vi "Formatdata.vi"() -> ()   [LabVIEW 2022 SP3, in "Switch_Keysight_34934A.lvlib" / "Switch_Keysight_34934A.lvclass"]
uses:
  Switch_Keysight_34934A.lvclass
  Components/ViPER.lvlibp/ViPER.lvclass
panel:
  in  "Config 2":T1={"VISA"="USB0::0x0957::0x0507::MY56485422::INSTR", "Slot"=1, "SwitchMap"=[{"Name"="Passive_Tests", "Route"=[], "UnRoute"=[], "Description"="Tests component values unpowered", "Group"="", "IsGroup"=TRUE}, {"Name"="Discharge_C108_C109", "Route"=["M1H:1:6:1", "M1H:1:19:1", "M1L:1:6:1", "M1L:1:19:1"], "UnRoute"=["M1H:1:6:0", "M1H:1:19:0", "M1L:1:6:0", "M1L:1:19:0"], "Description"="Discharge the caps for 3 secs", "Group"="Passive_Tests", "IsGroup"=FALSE}, {"Name"="Capacitors", "Route"=[], "UnRoute"=[], "Description"="Tests Capacitor Values", "Group"="Passive_Tests", "IsGroup"=TRUE}, {"Name"="Connect_LCR", "Route"=["M1H:1:23:1", "M1H:2:24:1", "M1L:1:25:1", "M1L:2:26:1"], "UnRoute"=["M1H:1:23:0", "M1H:2:24:0", "M1L:1:25:0", "M1L:2:26:0"], "Description"="Connect the LCR to the Matrix", "Group"="Capacitors", "IsGroup"=FALSE}, {"Name"="C108_C109", "Route"=["M1H:1:6:1", "M1H:2:6:1", "M1L:1:6:1", "M1L:2:6:1"], "UnRoute"=["M1H:1:6:0", "M1H:2:6:0", "M1L:1:6:0", "M1L:2:6:0"], "Description"="C108 and C109 to LCR", "Group"="Capacitors", "IsGroup"=FALSE}, {"Name"="C153", "Route"=["M1H:1:7:1", "M1H:2:7:1", "M1L:1:5:1", "M1L:2:5:1"], "UnRoute"=["M1H:1:7:0", "M1H:2:7:0", "M1L:1:5:0", "M1L:2:5:0"], "Description"="C153 to LCR", "Group"="Capacitors", "IsGroup"=FALSE}, {"Name"="C1300", "Route"=["M1H:1:2:1", "M1H:2:2:1", "M1L:1:7:1", "M1L:2:7:1"], "UnRoute"=["M1H:1:2:0", "M1H:2:2:0", "M1L:1:7:0", "M1L:2:7:0"], "Description"="C1300 to LCR", "Group"="Capacitors", "IsGroup"=FALSE}, {"Name"="C701", "Route"=["M1H:1:8:1", "M1H:2:8:1", "M1L:1:2:1", "M1L:2:2:1"], "UnRoute"=["M1H:1:8:0", "M1H:2:8:0", "M1L:1:2:0", "M1L:2:2:0"], "Description"="C701 to LCR", "Group"="Capacitors", "IsGroup"=FALSE}, {"Name"="C1202", "Route"=["M1H:1:2:1", "M1H:2:2:1", "M1L:1:8:1", "M1L:2:8:1"], "UnRoute"=["M1H:1:2:0", "M1H:2:2:0", "M1L:1:8:0", "M1L:2:8:0"], "Description"="C1202 to LCR", "Group"="Capacitors", "IsGroup"=FALSE}, {"Name"="C1204", "Route"=["M1H:1:9:1", "M1H:2:9:1", "M1L:1:2:1", "M1L:2:2:1"], "UnRoute"=["M1H:1:9:0", "M1H:2:9:0", "M1L:1:2:0", "M1L:2:2:0"], "Description"="C1204 to LCR", "Group"="Capacitors", "IsGroup"=FALSE}, {"Name"="C1200", "Route"=["M1H:1:2:1", "M1H:2:2:1", "M1L:1:9:1", "M1L:2:9:1"], "UnRoute"=["M1H:1:2:0", "M1H:2:2:0", "M1L:1:9:0", "M1L:2:9:0"], "Description"="C1200 to LCR", "Group"="Capacitors", "IsGroup"=FALSE}, {"Name"="Resistors", "Route"=[], "UnRoute"=[], "Description"="Connect resistances to the DMM", "Group"="Passive_Tests", "IsGroup"=TRUE}, {"Name"="24V_to_Gnd", "Route"=[], "UnRoute"=[], "Description"="Ensure supply is not short circuit", "Group"="Resistors", "IsGroup"=FALSE}, {"Name"="R121", "Route"=["M1H:1:3:1", "M1H:2:3:1", "M1H:3:5:1", "M1H:4:5:1"], "UnRoute"=["M1H:1:3:0", "M1H:2:3:0", "M1H:3:5:0", "M1H:4:5:0"], "Description"="R121 to DMM", "Group"="Resistors", "IsGroup"=FALSE}, {"Name"="LUG", "Route"=["M1H:1:10:1", "M1H:2:10:1", "M1H:3:2:1", "M1H:4:2:1"], "UnRoute"=["M1H:1:10:0", "M1H:2:10:0", "M1H:3:2:0", "M1H:4:2:0"], "Description"="LUG to DMM", "Group"="Resistors", "IsGroup"=FALSE}, {"Name"="R304", "Route"=["M1L:1:10:1", "M1L:2:10:1", "M1L:3:2:1", "M1L:4:2:1"], "UnRoute"=["M1L:1:10:0", "M1L:2:10:0", "M1L:3:2:0", "M1L:4:2:0"], "Description"="R304 to DMM", "Group"="Resistors", "IsGroup"=FALSE}, {"Name"="R203", "Route"=["M1H:1:11:1", "M1H:2:11:1", "M1L:3:11:1", "M1L:4:11:1"], "UnRoute"=["M1H:1:11:0", "M1H:2:11:0", "M1L:3:11:0", "M1L:4:11:0"], "Description"="R203 to DMM", "Group"="Resistors", "IsGroup"=FALSE}, {"Name"="R207", "Route"=["M1H:1:16:1", "M1H:2:16:1", "M1L:3:15:1", "M1L:4:15:1"], "UnRoute"=["M1H:1:16:0", "M1H:2:16:0", "M1L:3:15:0", "M1L:4:15:0"], "Description"="R207 to DMM", "Group"="Resistors", "IsGroup"=FALSE}, {"Name"="R200", "Route"=["M1H:1:3:1", "M1H:2:3:1", "M1L:3:16:1", "M1L:4:16:1"], "UnRoute"=["M1H:1:3:0", "M1H:2:3:0", "M1L:3:16:0", "M1L:4:16:0"], "Description"="R200 to DMM", "Group"="Resistors", "IsGroup"=FALSE}, {"Name"="R201", "Route"=["M1H:1:3:1", "M1H:2:3:1", "M1H:3:17:1", "M1H:4:17:1"], "UnRoute"=["M1H:1:3:0", "M1H:2:3:0", "M1H:3:17:0", "M1H:4:17:0"], "Description"="R201 to DMM", "Group"="Resistors", "IsGroup"=FALSE}, {"Name"="R215", "Route"=["M1L:1:12:1", "M1L:2:12:1", "M1L:3:2:1", "M1L:4:2:1"], "UnRoute"=["M1L:1:12:0", "M1L:2:12:0", "M1L:3:2:0", "M1L:4:2:0"], "Description"="R215 to DMM", "Group"="Resistors", "IsGroup"=FALSE}, {"Name"="R214", "Route"=["M1H:1:2:1", "M1H:2:2:1", "M1L:3:12:1", "M1L:4:12:1"], "UnRoute"=["M1H:1:2:0", "M1H:2:2:0", "M1L:3:12:0", "M1L:4:12:0"], "Description"="R214 to DMM", "Group"="Resistors", "IsGroup"=FALSE}, {"Name"="R412", "Route"=["M1L:1:3:1", "M1L:2:3:1", "M1L:3:17:1", "M1L:4:17:1"], "UnRoute"=["M1L:1:3:0", "M1L:2:3:0", "M1L:3:17:0", "M1L:4:17:0"], "Description"="R412 to DMM", "Group"="Resistors", "IsGroup"=FALSE}, {"Name"="R413", "Route"=["M1H:1:13:1", "M1H:2:13:1", "M1H:3:2:1", "M1H:4:2:1"], "UnRoute"=["M1H:1:13:0", "M1H:2:13:0", "M1H:3:2:0", "M1H:4:2:0"], "Description"="R413 to DMM", "Group"="Resistors", "IsGroup"=FALSE}, {"Name"="R416", "Route"=["M1L:1:13:1", "M1L:2:13:1", "M1L:3:2:1", "M1L:4:2:1"], "UnRoute"=["M1L:1:13:0", "M1L:2:13:0", "M1L:3:2:0", "M1L:4:2:0"], "Description"="R416 to DMM", "Group"="Resistors", "IsGroup"=FALSE}, {"Name"="SP500", "Route"=["M1H:1:14:1", "M1H:2:14:1", "M1H:3:18:1", "M1H:4:18:1"], "UnRoute"=["M1H:1:14:0", "M1H:2:14:0", "M1H:3:18:0", "M1H:4:18:0"], "Description"="SP500 to DMM", "Group"="Resistors", "IsGroup"=FALSE}, {"Name"="R1204", "Route"=["M1L:1:2:1", "M1L:2:2:1", "M1L:3:14:1", "M1L:4:14:1"], "UnRoute"=["M1L:1:2:0", "M1L:2:2:0", "M1L:3:14:0", "M1L:4:14:0"], "Description"="R1204 to DMM", "Group"="Resistors", "IsGroup"=FALSE}, {"Name"="R1205_R1206", "Route"=["M1H:1:15:1", "M1H:2:15:1", "M1L:3:18:1", "M1L:4:18:1"], "UnRoute"=["M1H:1:15:0", "M1H:2:15:0", "M1L:3:18:0", "M1L:4:18:0"], "Description"="R1205 and R1206 to DMM", "Group"="Resistors", "IsGroup"=FALSE}, {"Name"="Diodes", "Route"=[], "UnRoute"=[], "Description"="Connect Diodes to the DMM with PSU", "Group"="Passive_Tests", "IsGroup"=TRUE}, {"Name"="D1200", "Route"=["M1H:1:15:1", "M1H:3:2:1", "M1H:3:28:1", "M1L:2:18:1", "M1L:2:27:1"], "UnRoute"=["M1H:1:15:0", "M1H:3:2:0", "M1H:3:28:0", "M1L:2:18:0", "M1L:2:27:0"], "Description"="D1200 to DMM and PSU", "Group"="Diodes", "IsGroup"=FALSE}, {"Name"="Active_Tests", "Route"=[], "UnRoute"=[], "Description"="Tests under power", "Group"="", "IsGroup"=TRUE}, {"Name"="Voltages", "Route"=[], "UnRoute"=[], "Description"="Connect test points to DMM", "Group"="Active_Tests", "IsGroup"=TRUE}, {"Name"="V_CON_24VIN", "Route"=["M2H:1:2:1", "M2L:3:2:1"], "UnRoute"=["M2H:1:2:0", "M2L:3:2:0"], "Description"="24V line to DMM", "Group"="Voltages", "IsGroup"=FALSE}, {"Name"="V_CON_Power_Switch", "Route"=["M1H:1:6:1", "M1L:3:6:1"], "UnRoute"=["M1H:1:6:0", "M1L:3:6:0"], "Description"="Power Switch to DMM", "Group"="Voltages", "IsGroup"=FALSE}, {"Name"="V_PSU_24V", "Route"=["M2H:1:3:1", "M2H:3:1:1"], "UnRoute"=["M2H:1:3:0", "M2H:3:1:0"], "Description"="PSU 12V to DMM +ve", "Group"="Voltages", "IsGroup"=FALSE}, {"Name"="V_PSU_5V", "Route"=["M2H:1:4:1", "M2H:3:1:1"], "UnRoute"=["M2H:1:4:0", "M2H:3:1:0"], "Description"="PSU 5V to DMM +ve", "Group"="Voltages", "IsGroup"=FALSE}, {"Name"="V_PSU_3V3", "Route"=["M2L:1:4:1", "M2H:3:1:1"], "UnRoute"=["M2L:1:4:0", "M2H:3:1:0"], "Description"="PSU 3V3 to DMM +ve", "Group"="Voltages", "IsGroup"=FALSE}, {"Name"="V_PSU_AREF_2V5", "Route"=["M2H:1:5:1", "M2H:3:1:1"], "UnRoute"=["M2H:1:5:0", "M2H:3:1:0"], "Description"="PSU AREF 2V5 to DMM +ve", "Group"="Voltages", "IsGroup"=FALSE}, {"Name"="V_PSU_AREF_1V25", "Route"=["M2L:1:5:1", "M2H:3:1:1"], "UnRoute"=["M2L:1:5:0", "M2H:3:1:0"], "Description"="PSU AREF 1V25 to DMM +ve", "Group"="Voltages", "IsGroup"=FALSE}, {"Name"="V_PSU_4V8", "Route"=["M2H:1:6:1", "M2H:3:1:1"], "UnRoute"=["M2H:1:6:0", "M2H:3:1:0"], "Description"="PSU 4V8to DMM +ve", "Group"="Voltages", "IsGroup"=FALSE}, {"Name"="V_PSU_PWR_GOOD", "Route"=["M2H:1:6:1", "M2H:1:27:1", "M2H:3:28:1", "M2L:1:6:1", "M2H:3:1:1"], "UnRoute"=["M2H:1:6:0", "M2H:1:27:0", "M2H:3:28:0", "M2L:1:6:0", "M2H:3:1:0"], "Description"="Connects PWR GOOD to PSU and DMM", "Group"="Voltages", "IsGroup"=FALSE}, {"Name"="V_PSU_3V3_ANA", "Route"=["M2H:1:7:1", "M2H:3:1:1"], "UnRoute"=["M2H:1:7:0", "M2H:3:1:0"], "Description"="Connects PSU 3V3 ANA to DMM +ve", "Group"="Voltages", "IsGroup"=FALSE}, {"Name"="V_PSU_WDOG_STAT", "Route"=["M2H:1:7:1", "M2H:3:1:1"], "UnRoute"=["M2H:1:7:0", "M2H:3:1:0"], "Description"="Connects PSU WDOG STAT to DMM +ve", "Group"="Voltages", "IsGroup"=FALSE}, {"Name"="V_PSU_WDOG_24V", "Route"=["M2H:1:8:1", "M2H:3:1:1"], "UnRoute"=["M2H:1:8:0", "M2H:3:1:0"], "Description"="Connects PSU WDOG 24V to DMM +ve", "Group"="Voltages", "IsGroup"=FALSE}, {"Name"="V_Valve1", "Route"=["M2H:3:9:1", "M2H:1:8:1"], "UnRoute"=["M2H:3:9:0", "M2H:1:8:0"], "Description"="Valve1 to DMM", "Group"="Voltages", "IsGroup"=FALSE}, {"Name"="V_Valve2", "Route"=["M2L:3:9:1", "M2H:1:8:1"], "UnRoute"=["M2L:3:9:0", "M2H:1:8:0"], "Description"="Valve2 to DMM", "Group"="Voltages", "IsGroup"=FALSE}, {"Name"="V_Valve3", "Route"=["M2H:3:10:1", "M2H:1:8:1"], "UnRoute"=["M2H:3:10:0", "M2H:1:8:0"], "Description"="Valve3 to DMM", "Group"="Voltages", "IsGroup"=FALSE}, {"Name"="V_Valve4", "Route"=["M2H:3:11:1", "M2H:1:8:1"], "UnRoute"=["M2H:3:11:0", "M2H:1:8:0"], "Description"="Valve4 to DMM", "Group"="Voltages", "IsGroup"=FALSE}, {"Name"="V_Valve5", "Route"=["M2H:3:11:1", "M2H:1:8:1"], "UnRoute"=["M2H:3:11:0", "M2H:1:8:0"], "Description"="Valve5 to DMM", "Group"="Voltages", "IsGroup"=FALSE}, {"Name"="V_Valve6", "Route"=["M2L:3:11:1", "M2H:1:8:1"], "UnRoute"=["M2L:3:11:0", "M2H:1:8:0"], "Description"="Valve6 to DMM", "Group"="Voltages", "IsGroup"=FALSE}, {"Name"="V_Valve7", "Route"=["M2H:3:12:1", "M2H:1:8:1"], "UnRoute"=["M2H:3:12:0", "M2H:1:8:0"], "Description"="Valve7 to DMM", "Group"="Voltages", "IsGroup"=FALSE}, {"Name"="V_Valve8", "Route"=["M2L:3:12:1", "M2H:1:8:1"], "UnRoute"=["M2L:3:12:0", "M2H:1:8:0"], "Description"="Valve8 to DMM", "Group"="Voltages", "IsGroup"=FALSE}, {"Name"="V_ValveDrain", "Route"=["M2L:3:12:1", "M2H:1:8:1"], "UnRoute"=["M2L:3:12:0", "M2H:1:8:0"], "Description"="ValveDrain to DMM", "Group"="Voltages", "IsGroup"=FALSE}, {"Name"="V_ValveTemp", "Route"=["M2L:3:13:1", "M2H:1:8:1"], "UnRoute"=["M2L:3:13:0", "M2H:1:8:0"], "Description"="ValveTemp to DMM", "Group"="Voltages", "IsGroup"=FALSE}, {"Name"="V_ValvePump", "Route"=["M2H:3:14:1", "M2H:1:8:1"], "UnRoute"=["M2H:3:14:0", "M2H:1:8:0"], "Description"="ValvePump to DMM", "Group"="Voltages", "IsGroup"=FALSE}, {"Name"="V_ValveLarge", "Route"=["M2H:3:14:1", "M2H:1:8:1"], "UnRoute"=["M2H:3:14:0", "M2H:1:8:0"], "Description"="ValveLarge to DMM", "Group"="Voltages", "IsGroup"=FALSE}, {"Name"="V_ValveSmall", "Route"=["M2H:3:14:1", "M2H:1:8:1"], "UnRoute"=["M2H:3:14:0", "M2H:1:8:0"], "Description"="ValveSmall to DMM", "Group"="Voltages", "IsGroup"=FALSE}, {"Name"="V_ValvePV1", "Route"=["M2L:3:15:1", "M2H:1:8:1"], "UnRoute"=["M2L:3:15:0", "M2H:1:8:0"], "Description"="ValvePV1 to DMM", "Group"="Voltages", "IsGroup"=FALSE}, {"Name"="V_ValvePV2", "Route"=["M2H:3:16:1", "M2H:1:8:1"], "UnRoute"=["M2H:3:16:0", "M2H:1:8:0"], "Description"="ValvePV2 to DMM", "Group"="Voltages", "IsGroup"=FALSE}, {"Name"="V_Fan", "Route"=["M2L:3:16:1", "M2H:1:8:1"], "UnRoute"=["M2L:3:16:0", "M2H:1:8:0"], "Description"="Fan to DMM", "Group"="Voltages", "IsGroup"=FALSE}], "Sim"=TRUE}
  in  "xml string":string="<Config><NumElts>3</NumElts><Refnum><Name>VISA</Name><RefKind>VISA</RefKind><Val>USB0::0x0957::0x0507::MY56485422::INSTR</Val></Refnum><I32><Name>Slot</Name><Val>1</Val></I32><Array><Name>SwitchMap</Name><Dimsize>131</Dimsize><Cluster><Name>Alias</Name><NumElts>2</NumElts><String><Name>Name</Name><Val>null</Val></String><Array><Name>Route</Name><Dimsize>0</Dimsize><String><Name>String</Name><Val /></String></Array></Cluster><Cluster><Name>Alias</Name><NumElts>2</NumElts><String><Name>Name</Name><Val>boot_uSD</Val></String><Array><Name>Route</Name><Dimsize>2</Dimsize><String><Name>String</Name><Val>M1L:3:2:1</Val></String><String><Name>String</Name><Val>M1L:3:17:1</Val></String></Array></Cluster><Cluster><Name>Alias</Name><NumElts>2</NumElts><String><Name>Name</Name><Val>boot_eMMC</Val></String><Array><Name>Route</Name><Dimsize>2</Dimsize><String><Name>String</Name><Val>M1L:3:2:0</Val></String><String><Name>String</Name><Val>M1L:3:17:0</Val></String></Array></Cluster><Cluster><Name>Alias</Name><NumElts>2</NumElts><String><Name>Name</Name><Val>con_rs485_loopback</Val></String><Array><Name>Route</Name><Dimsize>4</Dimsize><String><Name>String</Name><Val>M1H:2:11:1</Val></String><String><Name>String</Name><Val>M1H:2:16:1</Val></String><String><Name>String</Name><Val>M1L:4:11:1</Val></String><String><Name>String</Name><Val>M1L:4:15:1</Val></String></Array></Cluster><Cluster><Name>Alias</Name><NumElts>2</NumElts><String><Name>Name</Name><Val>dis_rs485_loopback</Val></String><Array><Name>Route</Name><Dimsize>4</Dimsize><String><Name>String</Name><Val>M1H:2:11:0</Val></String><String><Name>String</Name><Val>M1H:2:16:0</Val></String><String><Name>String</Name><Val>M1L:4:11:0</Val></String><String><Name>String</Name><Val>M1L:4:15:0</Val></String></Array></Cluster><Cluster><Name>Alias</Name><NumElts>2</NumElts><String><Name>Name</Name><Val>con_discharge_c108_c109</Val></String><Array><Name>Route</Name><Dimsize>4</Dimsize><String><Name>String</Name><Val>M1H:1:6:1</Val></String><String><Name>String</Name><Val>M1H:1:19:1</Val></String><String><Name>String</Name><Val>M1L:1:6:1</Val></String><String><Name>String</Name><Val>M1L:1:19:1</Val></String></Array></Cluster><Cluster><Name>Alias</Name><NumElts>2</NumElts><String><Name>Name</Name><Val>dis_discharge_c108_c109</Val></String><Array><Name>Route</Name><Dimsize>4</Dimsize><String><Name>String</Name><Val>M1H:1:6:0</Val></String><String><Name>String</Name><Val>M1H:1:19:0</Val></String><String><Name>String</Name><Val>M1L:1:6:0</Val></String><String><Name>String</Name><Val>M1L:1:19:0</Val></String></Array></Cluster><Cluster><Name>Alias</Name><NumElts>2</NumElts><String><Name>Name</Name><Val>con_lcr</Val></String><Array><Name>Route</Name><Dimsize>4</Dimsize><String><Name>String</Name><Val>M1H:1:23:1</Val></String><String><Name>String</Name><Val>M1H:2:24:1</Val></String><String><Name>String</Name><Val>M1L:1:25:1</Val></String><String><Name>String</Name><Val>M1L:2:26:1</Val></String></Array></Cluster><Cluster><Name>Alias</Name><NumElts>2</NumElts><String><Name>Name</Name><Val>dis_lcr</Val></String><Array><Name>Route</Name><Dimsize>4</Dimsize><String><Name>String</Name><Val>M1H:1:23:0</Val></String><String><Name>String</Name><Val>M1H:2:24:0</Val></String><String><Name>String</Name><Val>M1L:1:25:0</Val></String><String><Name>String</Name><Val>M1L:2:26:0</Val></String></Array></Cluster><Cluster><Name>Alias</Name><NumElts>2</NumElts><String><Name>Name</Name><Val>con_c108_c109</Val></String><Array><Name>Route</Name><Dimsize>4</Dimsize><String><Name>String</Name><Val>M1H:1:6:1</Val></String><String><Name>String</Name><Val>M1H:2:6:1</Val></String><String><Name>String</Name><Val>M1L:1:6:1</Val></String><String><Name>String</Name><Val>M1L:2:6:1</Val></String></Array></Cluster><Cluster><Name>Alias</Name><NumElts>2</NumElts><String><Name>Name</Name><Val>dis_c108_c109</Val></String><Array><Name>Route</Name><Dimsize>4</Dimsize><String><Name>String</Name><Val>M1H:1:6:0</Val></String><String><Name>String</Name><Val>M1H:2:6:0</Val></String><String><Name>String</Name><Val>M1L:1:6:0</Val></String><String><Name>String</Name><Val>M1L:2:6:0</Val></String></Array></Cluster><Cluster><Name>Alias</Name><NumElts>2</NumElts><String><Name>Name</Name><Val>con_c153</Val></String><Array><Name>Route</Name><Dimsize>4</Dimsize><String><Name>String</Name><Val>M1H:1:7:1</Val></String><String><Name>String</Name><Val>M1H:2:7:1</Val></String><String><Name>String</Name><Val>M1L:1:5:1</Val></String><String><Name>String</Name><Val>M1L:2:5:1</Val></String></Array></Cluster><Cluster><Name>Alias</Name><NumElts>2</NumElts><String><Name>Name</Name><Val>dis_c153</Val></String><Array><Name>Route</Name><Dimsize>4</Dimsize><String><Name>String</Name><Val>M1H:1:7:0</Val></String><String><Name>String</Name><Val>M1H:2:7:0</Val></String><String><Name>String</Name><Val>M1L:1:5:0</Val></String><String><Name>String</Name><Val>M1L:2:5:0</Val></String></Array></Cluster><Cluster><Name>Alias</Name><NumElts>2</NumElts><String><Name>Name</Name><Val>con_c1300</Val></String><Array><Name>Route</Name><Dimsize>4</Dimsize><String><Name>String</Name><Val>M1H:1:2:1</Val></String><String><Name>String</Name><Val>M1H:2:2:1</Val></String><String><Name>String</Name><Val>M1L:1:7:1</Val></String><String><Name>String</Name><Val>M1L:2:7:1</Val></String></Array></Cluster><Cluster><Name>Alias</Name><NumElts>2</NumElts><String><Name>Name</Name><Val>dis_c1300</Val></String><Array><Name>Route</Name><Dimsize>4</Dimsize><String><Name>String</Name><Val>M1H:1:2:0</Val></String><String><Name>String</Name><Val>M1H:2:2:0</Val></String><String><Name>String</Name><Val>M1L:1:7:0</Val></String><String><Name>String</Name><Val>M1L:2:7:0</Val></String></Array></Cluster><Cluster><Name>Alias</Name><NumElts>2</NumElts><String><Name>Name</Name><Val>con_c701</Val></String><Array><Name>Route</Name><Dimsize>4</Dimsize><String><Name>String</Name><Val>M1H:1:8:1</Val></String><String><Name>String</Name><Val>M1H:2:8:1</Val></String><String><Name>String</Name><Val>M1L:1:2:1</Val></String><String><Name>String</Name><Val>M1L:2:2:1</Val></String></Array></Cluster><Cluster><Name>Alias</Name><NumElts>2</NumElts><String><Name>Name</Name><Val>dis_c701</Val></String><Array><Name>Route</Name><Dimsize>4</Dimsize><String><Name>String</Name><Val>M1H:1:8:0</Val></String><String><Name>String</Name><Val>M1H:2:8:0</Val></String><String><Name>String</Name><Val>M1L:1:2:0</Val></String><String><Name>String</Name><Val>M1L:2:2:0</Val></String></Array></Cluster><Cluster><Name>Alias</Name><NumElts>2</NumElts><String><Name>Name</Name><Val>con_c1202</Val></String><Array><Name>Route</Name><Dimsize>4</Dimsize><String><Name>String</Name><Val>M1H:1:2:1</Val></String><String><Name>String</Name><Val>M1H:2:2:1</Val></String><String><Name>String</Name><Val>M1L:1:8:1</Val></String><String><Name>String</Name><Val>M1L:2:8:1</Val></String></Array></Cluster><Cluster><Name>Alias</Name><NumElts>2</NumElts><String><Name>Name</Name><Val>dis_c1202</Val></String><Array><Name>Route</Name><Dimsize>4</Dimsize><String><Name>String</Name><Val>M1H:1:2:0</Val></String><String><Name>String</Name><Val>M1H:2:2:0</Val></String><String><Name>String</Name><Val>M1L:1:8:0</Val></String><String><Name>String</Name><Val>M1L:2:8:0</Val></String></Array></Cluster><Cluster><Name>Alias</Name><NumElts>2</NumElts><String><Name>Name</Name><Val>con_c1204</Val></String><Array><Name>Route</Name><Dimsize>4</Dimsize><String><Name>String</Name><Val>M1H:1:9:1</Val></String><String><Name>String</Name><Val>M1H:2:9:1</Val></String><String><Name>String</Name><Val>M1L:1:2:1</Val></String><String><Name>String</Name><Val>M1L:2:2:1</Val></String></Array></Cluster><Cluster><Name>Alias</Name><NumElts>2</NumElts><String><Name>Name</Name><Val>dis_c1204</Val></String><Array><Name>Route</Name><Dimsize>4</Dimsize><String><Name>String</Name><Val>M1H:1:9:0</Val></String><String><Name>String</Name><Val>M1H:2:9:0</Val></String><String><Name>String</Name><Val>M1L:1:2:0</Val></String><String><Name>String</Name><Val>M1L:2:2:0</Val></String></Array></Cluster><Cluster><Name>Alias</Name><NumElts>2</NumElts><String><Name>Name</Name><Val>con_c1200</Val></String><Array><Name>Route</Name><Dimsize>4</Dimsize><String><Name>String</Name><Val>M1H:1:2:1</Val></String><String><Name>String</Name><Val>M1H:2:2:1</Val></String><String><Name>String</Name><Val>M1L:1:9:1</Val></String><String><Name>String</Name><Val>M1L:2:9:1</Val></String></Array></Cluster><Cluster><Name>Alias</Name><NumElts>2</NumElts><String><Name>Name</Name><Val>dis_c1200</Val></String><Array><Name>Route</Name><Dimsize>4</Dimsize><String><Name>String</Name><Val>M1H:1:2:0</Val></String><String><Name>String</Name><Val>M1H:2:2:0</Val></String><String><Name>String</Name><Val>M1L:1:9:0</Val></String><String><Name>String</Name><Val>M1L:2:9:0</Val></String></Array></Cluster><Cluster><Name>Alias</Name><NumElts>2</NumElts><String><Name>Name</Name><Val>con_24v_to_gnd</Val></String><Array><Name>Route</Name><Dimsize>4</Dimsize><String><Name>String</Name><Val>M2H:1:3:1</Val></String><String><Name>String</Name><Val>M2H:2:3:1</Val></String><String><Name>String</Name><Val>M2L:3:1:1</Val></String><String><Name>String</Name><Val>M2L:4:1:1</Val></String></Array></Cluster><Cluster><Name>Alias</Name><NumElts>2</NumElts><String><Name>Name</Name><Val>dis_24v_to_gnd</Val></String><Array><Name>Route</Name><Dimsize>4</Dimsize><String><Name>String</Name><Val>M2H:1:3:0</Val></String><String><Name>String</Name><Val>M2H:2:3:0</Val></String><String><Name>String</Name><Val>M2L:3:1:0</Val></String><String><Name>String</Name><Val>M2L:4:1:0</Val></String></Array></Cluster><Cluster><Name>Alias</Name><NumElts>2</NumElts><String><Name>Name</Name><Val>con_r121</Val></String><Array><Name>Route</Name><Dimsize>4</Dimsize><String><Name>String</Name><Val>M1H:1:3:1</Val></String><String><Name>String</Name><Val>M1H:2:3:1</Val></String><String><Name>String</Name><Val>M1H:3:5:1</Val></String><String><Name>String</Name><Val>M1H:4:5:1</Val></String></Array></Cluster><Cluster><Name>Alias</Name><NumElts>2</NumElts><String><Name>Name</Name><Val>dis_r121</Val></String><Array><Name>Route</Name><Dimsize>4</Dimsize><String><Name>String</Name><Val>M1H:1:3:0</Val></String><String><Name>String</Name><Val>M1H:2:3:0</Val></String><String><Name>String</Name><Val>M1H:3:5:0</Val></String><String><Name>String</Name><Val>M1H:4:5:0</Val></String></Array></Cluster><Cluster><Name>Alias</Name><NumElts>2</NumElts><String><Name>Name</Name><Val>con_lug</Val></String><Array><Name>Route</Name><Dimsize>4</Dimsize><String><Name>String</Name><Val>M1H:1:10:1</Val></String><String><Name>String</Name><Val>M1H:2:10:1</Val></String><String><Name>String</Name><Val>M1H:3:2:1</Val></String><String><Name>String</Name><Val>M1H:4:2:1</Val></String></Array></Cluster><Cluster><Name>Alias</Name><NumElts>2</NumElts><String><Name>Name</Name><Val>dis_lug</Val></String><Array><Name>Route</Name><Dimsize>4</Dimsize><String><Name>String</Name><Val>M1H:1:10:0</Val></String><String><Name>String</Name><Val>M1H:2:10:0</Val></String><String><Name>String</Name><Val>M1H:3:2:0</Val></String><String><Name>String</Name><Val>M1H:4:2:0</Val></String></Array></Cluster><Cluster><Name>Alias</Name><NumElts>2</NumElts><String><Name>Name</Name><Val>con_r304</Val></String><Array><Name>Route</Name><Dimsize>4</Dimsize><String><Name>String</Name><Val>M1L:1:10:1</Val></String><String><Name>String</Name><Val>M1L:2:10:1</Val></String><String><Name>String</Name><Val>M1L:3:2:1</Val></String><String><Name>String</Name><Val>M1L:4:2:1</Val></String></Array></Cluster><Cluster><Name>Alias</Name><NumElts>2</NumElts><String><Name>Name</Name><Val>dis_r304</Val></String><Array><Name>Route</Name><Dimsize>4</Dimsize><String><Name>String</Name><Val>M1L:1:10:0</Val></String><String><Name>String</Name><Val>M1L:2:10:0</Val></String><String><Name>String</Name><Val>M1L:3:2:0</Val></String><String><Name>String</Name><Val>M1L:4:2:0</Val></String></Array></Cluster><Cluster><Name>Alias</Name><NumElts>2</NumElts><String><Name>Name</Name><Val>con_r203</Val></String><Array><Name>Route</Name><Dimsize>4</Dimsize><String><Name>String</Name><Val>M1H:1:11:1</Val></String><String><Name>String</Name><Val>M1H:2:11:1</Val></String><String><Name>String</Name><Val>M1L:3:11:1</Val></String><String><Name>String</Name><Val>M1L:4:11:1</Val></String></Array></Cluster><Cluster><Name>Alias</Name><NumElts>2</NumElts><String><Name>Name</Name><Val>dis_r203</Val></String><Array><Name>Route</Name><Dimsize>4</Dimsize><String><Name>String</Name><Val>M1H:1:11:0</Val></String><String><Name>String</Name><Val>M1H:2:11:0</Val></String><String><Name>String</Name><Val>M1L:3:11:0</Val></String><String><Name>String</Name><Val>M1L:4:11:0</Val></String></Array></Cluster><Cluster><Name>Alias</Name><NumElts>2</NumElts><String><Name>Name</Name><Val>con_r207</Val></String><Array><Name>Route</Name><Dimsize>4</Dimsize><String><Name>String</Name><Val>M1H:1:16:1</Val></String><String><Name>String</Name><Val>M1H:2:16:1</Val></String><String><Name>String</Name><Val>M1L:3:15:1</Val></String><String><Name>String</Name><Val>M1L:4:15:1</Val></String></Array></Cluster><Cluster><Name>Alias</Name><NumElts>2</NumElts><String><Name>Name</Name><Val>dis_r207</Val></String><Array><Name>Route</Name><Dimsize>4</Dimsize><String><Name>String</Name><Val>M1H:1:16:0</Val></String><String><Name>String</Name><Val>M1H:2:16:0</Val></String><String><Name>String</Name><Val>M1L:3:15:0</Val></String><String><Name>String</Name><Val>M1L:4:15:0</Val></String></Array></Cluster><Cluster><Name>Alias</Name><NumElts>2</NumElts><String><Name>Name</Name><Val>con_r200</Val></String><Array><Name>Route</Name><Dimsize>4</Dimsize><String><Name>String</Name><Val>M1H:1:3:1</Val></String><String><Name>String</Name><Val>M1H:2:3:1</Val></String><String><Name>String</Name><Val>M1L:3:16:1</Val></String><String><Name>String</Name><Val>M1L:4:16:1</Val></String></Array></Cluster><Cluster><Name>Alias</Name><NumElts>2</NumElts><String><Name>Name</Name><Val>dis_r200</Val></String><Array><Name>Route</Name><Dimsize>4</Dimsize><String><Name>String</Name><Val>M1H:1:3:0</Val></String><String><Name>String</Name><Val>M1H:2:3:0</Val></String><String><Name>String</Name><Val>M1L:3:16:0</Val></String><String><Name>String</Name><Val>M1L:4:16:0</Val></String></Array></Cluster><Cluster><Name>Alias</Name><NumElts>2</NumElts><String><Name>Name</Name><Val>con_r201</Val></String><Array><Name>Route</Name><Dimsize>4</Dimsize><String><Name>String</Name><Val>M1H:1:3:1</Val></String><String><Name>String</Name><Val>M1H:2:3:1</Val></String><String><Name>String</Name><Val>M1H:3:17:1</Val></String><String><Name>String</Name><Val>M1H:4:17:1</Val></String></Array></Cluster><Cluster><Name>Alias</Name><NumElts>2</NumElts><String><Name>Name</Name><Val>dis_r201</Val></String><Array><Name>Route</Name><Dimsize>4</Dimsize><String><Name>String</Name><Val>M1H:1:3:0</Val></String><String><Name>String</Name><Val>M1H:2:3:0</Val></String><String><Name>String</Name><Val>M1H:3:17:0</Val></String><String><Name>String</Name><Val>M1H:4:17:0</Val></String></Array></Cluster><Cluster><Name>Alias</Name><NumElts>2</NumElts><String><Name>Name</Name><Val>con_r215</Val></String><Array><Name>Route</Name><Dimsize>4</Dimsize><String><Name>String</Name><Val>M1L:1:12:1</Val></String><String><Name>String</Name><Val>M1L:2:12:1</Val></String><String><Name>String</Name><Val>M1L:3:2:1</Val></String><String><Name>String</Name><Val>M1L:4:2:1</Val></String></Array></Cluster><Cluster><Name>Alias</Name><NumElts>2</NumElts><String><Name>Name</Name><Val>dis_r215</Val></String><Array><Name>Route</Name><Dimsize>4</Dimsize><String><Name>String</Name><Val>M1L:1:12:0</Val></String><String><Name>String</Name><Val>M1L:2:12:0</Val></String><String><Name>String</Name><Val>M1L:3:2:0</Val></String><String><Name>String</Name><Val>M1L:4:2:0</Val></String></Array></Cluster><Cluster><Name>Alias</Name><NumElts>2</NumElts><String><Name>Name</Name><Val>con_r214</Val></String><Array><Name>Route</Name><Dimsize>4</Dimsize><String><Name>String</Name><Val>M1H:1:2:1</Val></String><String><Name>String</Name><Val>M1H:2:2:1</Val></String><String><Name>String</Name><Val>M1L:3:12:1</Val></String><String><Name>String</Name><Val>M1L:4:12:1</Val></String></Array></Cluster><Cluster><Name>Alias</Name><NumElts>2</NumElts><String><Name>Name</Name><Val>dis_r214</Val></String><Array><Name>Route</Name><Dimsize>4</Dimsize><String><Name>String</Name><Val>M1H:1:2:0</Val></String><String><Name>String</Name><Val>M1H:2:2:0</Val></String><String><Name>String</Name><Val>M1L:3:12:0</Val></String><String><Name>String</Name><Val>M1L:4:12:0</Val></String></Array></Cluster><Cluster><Name>Alias</Name><NumElts>2</NumElts><String><Name>Name</Name><Val>con_r412</Val></String><Array><Name>Route</Name><Dimsize>4</Dimsize><String><Name>String</Name><Val>M1L:1:3:1</Val></String><String><Name>String</Name><Val>M1L:2:3:1</Val></String><String><Name>String</Name><Val>M1L:3:17:1</Val></String><String><Name>String</Name><Val>M1L:4:17:1</Val></String></Array></Cluster><Cluster><Name>Alias</Name><NumElts>2</NumElts><String><Name>Name</Name><Val>dis_r412</Val></String><Array><Name>Route</Name><Dimsize>4</Dimsize><String><Name>String</Name><Val>M1L:1:3:0</Val></String><String><Name>String</Name><Val>M1L:2:3:0</Val></String><String><Name>String</Name><Val>M1L:3:17:0</Val></String><String><Name>String</Name><Val>M1L:4:17:0</Val></String></Array></Cluster><Cluster><Name>Alias</Name><NumElts>2</NumElts><String><Name>Name</Name><Val>con_413</Val></String><Array><Name>Route</Name><Dimsize>4</Dimsize><String><Name>String</Name><Val>M1H:1:13:1</Val></String><String><Name>String</Name><Val>M1H:2:13:1</Val></String><String><Name>String</Name><Val>M1H:3:2:1</Val></String><String><Name>String</Name><Val>M1H:4:2:1</Val></String></Array></Cluster><Cluster><Name>Alias</Name><NumElts>2</NumElts><String><Name>Name</Name><Val>dis_413</Val></String><Array><Name>Route</Name><Dimsize>4</Dimsize><String><Name>String</Name><Val>M1H:1:13:0</Val></String><String><Name>String</Name><Val>M1H:2:13:0</Val></String><String><Name>String</Name><Val>M1H:3:2:0</Val></String><String><Name>String</Name><Val>M1H:4:2:0</Val></String></Array></Cluster><Cluster><Name>Alias</Name><NumElts>2</NumElts><String><Name>Name</Name><Val>con_r416</Val></String><Array><Name>Route</Name><Dimsize>4</Dimsize><String><Name>String</Name><Val>M1L:1:13:1</Val></String><String><Name>String</Name><Val>M1L:2:13:1</Val></String><String><Name>String</Name><Val>M1L:3:2:1</Val></String><String><Name>String</Name><Val>M1L:4:2:1</Val></String></Array></Cluster><Cluster><Name>Alias</Name><NumElts>2</NumElts><String><Name>Name</Name><Val>dis_r416</Val></String><Array><Name>Route</Name><Dimsize>4</Dimsize><String><Name>String</Name><Val>M1L:1:13:0</Val></String><String><Name>String</Name><Val>M1L:2:13:0</Val></String><String><Name>String</Name><Val>M1L:3:2:0</Val></String><String><Name>String</Name><Val>M1L:4:2:0</Val></String></Array></Cluster><Cluster><Name>Alias</Name><NumElts>2</NumElts><String><Name>Name</Name><Val>con_sp500</Val></String><Array><Name>Route</Name><Dimsize>4</Dimsize><String><Name>String</Name><Val>M1H:1:14:1</Val></String><String><Name>String</Name><Val>M1H:2:14:1</Val></String><String><Name>String</Name><Val>M1H:3:18:1</Val></String><String><Name>String</Name><Val>M1H:4:18:1</Val></String></Array></Cluster><Cluster><Name>Alias</Name><NumElts>2</NumElts><String><Name>Name</Name><Val>dis_sp500</Val></String><Array><Name>Route</Name><Dimsize>4</Dimsize><String><Name>String</Name><Val>M1H:1:14:0</Val></String><String><Name>String</Name><Val>M1H:2:14:0</Val></String><String><Name>String</Name><Val>M1H:3:18:0</Val></String><String><Name>String</Name><Val>M1H:4:18:0</Val></String></Array></Cluster><Cluster><Name>Alias</Name><NumElts>2</NumElts><String><Name>Name</Name><Val>con_r1204</Val></String><Array><Name>Route</Name><Dimsize>4</Dimsize><String><Name>String</Name><Val>M1L:1:2:1</Val></String><String><Name>String</Name><Val>M1L:2:2:1</Val></String><String><Name>String</Name><Val>M1L:3:14:1</Val></String><String><Name>String</Name><Val>M1L:4:14:1</Val></String></Array></Cluster><Cluster><Name>Alias</Name><NumElts>2</NumElts><String><Name>Name</Name><Val>dis_r1204</Val></String><Array><Name>Route</Name><Dimsize>4</Dimsize><String><Name>String</Name><Val>M1L:1:2:0</Val></String><String><Name>String</Name><Val>M1L:2:2:0</Val></String><String><Name>String</Name><Val>M1L:3:14:0</Val></String><String><Name>String</Name><Val>M1L:4:14:0</Val></String></Array></Cluster><Cluster><Name>Alias</Name><NumElts>2</NumElts><String><Name>Name</Name><Val>con_r1205_r1206</Val></String><Array><Name>Route</Name><Dimsize>4</Dimsize><String><Name>String</Name><Val>M1H:1:15:1</Val></String><String><Name>String</Name><Val>M1H:2:15:1</Val></String><String><Name>String</Name><Val>M1L:3:18:1</Val></String><String><Name>String</Name><Val>M1L:4:18:1</Val></String></Array></Cluster><Cluster><Name>Alias</Name><NumElts>2</NumElts><String><Name>Name</Name><Val>dis_r1205_r1206</Val></String><Array><Name>Route</Name><Dimsize>4</Dimsize><String><Name>String</Name><Val>M1H:1:15:0</Val></String><String><Name>String</Name><Val>M1H:2:15:0</Val></String><String><Name>String</Name><Val>M1L:3:18:0</Val></String><String><Name>String</Name><Val>M1L:4:18:0</Val></String></Array></Cluster><Cluster><Name>Alias</Name><NumElts>2</NumElts><String><Name>Name</Name><Val>con_D1200</Val></String><Array><Name>Route</Name><Dimsize>5</Dimsize><String><Name>String</Name><Val>M1H:1:15:1</Val></String><String><Name>String</Name><Val>M1H:3:2:1</Val></String><String><Name>String</Name><Val>M1H:3:28:1</Val></String><String><Name>String</Name><Val>M1L:2:18:1</Val></String><String><Name>String</Name><Val>M1L:2:27:1</Val></String></Array></Cluster><Cluster><Name>Alias</Name><NumElts>2</NumElts><String><Name>Name</Name><Val>dis_D1200</Val></String><Array><Name>Route</Name><Dimsize>5</Dimsize><String><Name>String</Name><Val>M1H:1:15:0</Val></String><String><Name>String</Name><Val>M1H:3:2:0</Val></String><String><Name>String</Name><Val>M1H:3:28:0</Val></String><String><Name>String</Name><Val>M1L:2:18:0</Val></String><String><Name>String</Name><Val>M1L:2:27:0</Val></String></Array></Cluster><Cluster><Name>Alias</Name><NumElts>2</NumElts><String><Name>Name</Name><Val>con_24VIN</Val></String><Array><Name>Route</Name><Dimsize>2</Dimsize><String><Name>String</Name><Val>M2H:1:2:1</Val></String><String><Name>String</Name><Val>M2L:3:2:1</Val></String></Array></Cluster><Cluster><Name>Alias</Name><NumElts>2</NumElts><String><Name>Name</Name><Val>dis_24VIN</Val></String><Array><Name>Route</Name><Dimsize>2</Dimsize><String><Name>String</Name><Val>M2H:1:2:0</Val></String><String><Name>String</Name><Val>M2L:3:2:0</Val></String></Array></Cluster><Cluster><Name>Alias</Name><NumElts>2</NumElts><String><Name>Name</Name><Val>con_power_switch</Val></String><Array><Name>Route</Name><Dimsize>2</Dimsize><String><Name>String</Name><Val>M1H:1:6:1</Val></String><String><Name>String</Name><Val>M1L:3:6:1</Val></String></Array></Cluster><Cluster><Name>Alias</Name><NumElts>2</NumElts><String><Name>Name</Name><Val>dis_power_switch</Val></String><Array><Name>Route</Name><Dimsize>2</Dimsize><String><Name>String</Name><Val>M1H:1:6:0</Val></String><String><Name>String</Name><Val>M1L:3:6:0</Val></String></Array></Cluster><Cluster><Name>Alias</Name><NumElts>2</NumElts><String><Name>Name</Name><Val>con_gnd</Val></String><Array><Name>Route</Name><Dimsize>1</Dimsize><String><Name>String</Name><Val>M2H:3:1:1</Val></String></Array></Cluster><Cluster><Name>Alias</Name><NumElts>2</NumElts><String><Name>Name</Name><Val>dis_gnd</Val></String><Array><Name>Route</Name><Dimsize>1</Dimsize><String><Name>String</Name><Val>M2H:3:1:0</Val></String></Array></Cluster><Cluster><Name>Alias</Name><NumElts>2</NumElts><String><Name>Name</Name><Val>con_psu_24v</Val></String><Array><Name>Route</Name><Dimsize>1</Dimsize><String><Name>String</Name><Val>M2H:1:3:1</Val></String></Array></Cluster><Cluster><Name>Alias</Name><NumElts>2</NumElts><String><Name>Name</Name><Val>dis_psu_24v</Val></String><Array><Name>Route</Name><Dimsize>1</Dimsize><String><Name>String</Name><Val>M2H:1:3:0</Val></String></Array></Cluster><Cluster><Name>Alias</Name><NumElts>2</NumElts><String><Name>Name</Name><Val>con_psu_12v</Val></String><Array><Name>Route</Name><Dimsize>1</Dimsize><String><Name>String</Name><Val>M2L:1:3:1</Val></String></Array></Cluster><Cluster><Name>Alias</Name><NumElts>2</NumElts><String><Name>Name</Name><Val>dis_psu_12v</Val></String><Array><Name>Route</Name><Dimsize>1</Dimsize><String><Name>String</Name><Val>M2L:1:3:0</Val></String></Array></Cluster><Cluster><Name>Alias</Name><NumElts>2</NumElts><String><Name>Name</Name><Val>con_psu_5v</Val></String><Array><Name>Route</Name><Dimsize>1</Dimsize><String><Name>String</Name><Val>M2H:1:4:1</Val></String></Array></Cluster><Cluster><Name>Alias</Name><NumElts>2</NumElts><String><Name>Name</Name><Val>dis_psu_5v</Val></String><Array><Name>Route</Name><Dimsize>1</Dimsize><String><Name>String</Name><Val>M2H:1:4:0</Val></String></Array></Cluster><Cluster><Name>Alias</Name><NumElts>2</NumElts><String><Name>Name</Name><Val>con_psu_3v3</Val></String><Array><Name>Route</Name><Dimsize>1</Dimsize><String><Name>String</Name><Val>M2L:1:4:1</Val></String></Array></Cluster><Cluster><Name>Alias</Name><NumElts>2</NumElts><String><Name>Name</Name><Val>dis_psu_3v3</Val></String><Array><Name>Route</Name><Dimsize>1</Dimsize><String><Name>String</Name><Val>M2L:1:4:0</Val></String></Array></Cluster><Cluster><Name>Alias</Name><NumElts>2</NumElts><String><Name>Name</Name><Val>con_psu_aref_2v5</Val></String><Array><Name>Route</Name><Dimsize>1</Dimsize><String><Name>String</Name><Val>M2H:1:5:1</Val></String></Array></Cluster><Cluster><Name>Alias</Name><NumElts>2</NumElts><String><Name>Name</Name><Val>dis_psu_aref_2v5</Val></String><Array><Name>Route</Name><Dimsize>1</Dimsize><String><Name>String</Name><Val>M2H:1:5:0</Val></String></Array></Cluster><Cluster><Name>Alias</Name><NumElts>2</NumElts><String><Name>Name</Name><Val>con_psu_aref_1v25</Val></String><Array><Name>Route</Name><Dimsize>1</Dimsize><String><Name>String</Name><Val>M2L:1:5:1</Val></String></Array></Cluster><Cluster><Name>Alias</Name><NumElts>2</NumElts><String><Name>Name</Name><Val>dis_psu_aref_1v25</Val></String><Array><Name>Route</Name><Dimsize>1</Dimsize><String><Name>String</Name><Val>M2L:1:5:0</Val></String></Array></Cluster><Cluster><Name>Alias</Name><NumElts>2</NumElts><String><Name>Name</Name><Val>con_psu_4.8v</Val></String><Array><Name>Route</Name><Dimsize>1</Dimsize><String><Name>String</Name><Val>M2H:1:6:1</Val></String></Array></Cluster><Cluster><Name>Alias</Name><NumElts>2</NumElts><String><Name>Name</Name><Val>dis_psu_4.8v</Val></String><Array><Name>Route</Name><Dimsize>1</Dimsize><String><Name>String</Name><Val>M2H:1:6:0</Val></String></Array></Cluster><Cluster><Name>Alias</Name><NumElts>2</NumElts><String><Name>Name</Name><Val>con_psu_pwr_good</Val></String><Array><Name>Route</Name><Dimsize>4</Dimsize><String><Name>String</Name><Val>M2H:1:6:1</Val></String><String><Name>String</Name><Val>M2H:1:27:1</Val></String><String><Name>String</Name><Val>M2H:3:28:1</Val></String><String><Name>String</Name><Val>M2L:1:6:1</Val></String></Array></Cluster><Cluster><Name>Alias</Name><NumElts>2</NumElts><String><Name>Name</Name><Val>dis_psu_pwr_good</Val></String><Array><Name>Route</Name><Dimsize>4</Dimsize><String><Name>String</Name><Val>M2H:1:6:0</Val></String><String><Name>String</Name><Val>M2H:1:27:0</Val></String><String><Name>String</Name><Val>M2H:3:28:0</Val></String><String><Name>String</Name><Val>M2L:1:6:0</Val></String></Array></Cluster><Cluster><Name>Alias</Name><NumElts>2</NumElts><String><Name>Name</Name><Val>con_psu_3v3_ana</Val></String><Array><Name>Route</Name><Dimsize>1</Dimsize><String><Name>String</Name><Val>M2H:1:7:1</Val></String></Array></Cluster><Cluster><Name>Alias</Name><NumElts>2</NumElts><String><Name>Name</Name><Val>dis_psu_3v3_ana</Val></String><Array><Name>Route</Name><Dimsize>1</Dimsize><String><Name>String</Name><Val>M2H:1:7:0</Val></String></Array></Cluster><Cluster><Name>Alias</Name><NumElts>2</NumElts><String><Name>Name</Name><Val>con_wdog_stat</Val></String><Array><Name>Route</Name><Dimsize>1</Dimsize><String><Name>String</Name><Val>M2L:1:7:1</Val></String></Array></Cluster><Cluster><Name>Alias</Name><NumElts>2</NumElts><String><Name>Name</Name><Val>dis_wdog_stat</Val></String><Array><Name>Route</Name><Dimsize>1</Dimsize><String><Name>String</Name><Val>M2L:1:7:0</Val></String></Array></Cluster><Cluster><Name>Alias</Name><NumElts>2</NumElts><String><Name>Name</Name><Val>con_wdog_24v</Val></String><Array><Name>Route</Name><Dimsize>1</Dimsize><String><Name>String</Name><Val>M2H:1:8:1</Val></String></Array></Cluster><Cluster><Name>Alias</Name><NumElts>2</NumElts><String><Name>Name</Name><Val>dis_wdog_24v</Val></String><Array><Name>Route</Name><Dimsize>1</Dimsize><String><Name>String</Name><Val>M2H:1:8:0</Val></String></Array></Cluster><Cluster><Name>Alias</Name><NumElts>2</NumElts><String><Name>Name</Name><Val>con_tp140</Val></String><Array><Name>Route</Name><Dimsize>1</Dimsize><String><Name>String</Name><Val>M2H:1:8:1</Val></String></Array></Cluster><Cluster><Name>Alias</Name><NumElts>2</NumElts><String><Name>Name</Name><Val>dis_tp140</Val></String><Array><Name>Route</Name><Dimsize>1</Dimsize><String><Name>String</Name><Val>M2H:1:8:0</Val></String></Array></Cluster><Cluster><Name>Alias</Name><NumElts>2</NumElts><String><Name>Name</Name><Val>con_valve1</Val></String><Array><Name>Route</Name><Dimsize>1</Dimsize><String><Name>String</Name><Val>M2H:3:9:1</Val></String></Array></Cluster><Cluster><Name>Alias</Name><NumElts>2</NumElts><String><Name>Name</Name><Val>dis_valve1</Val></String><Array><Name>Route</Name><Dimsize>1</Dimsize><String><Name>String</Name><Val>M2H:3:9:0</Val></String></Array></Cluster><Cluster><Name>Alias</Name><NumElts>2</NumElts><String><Name>Name</Name><Val>con_valve2</Val></String><Array><Name>Route</Name><Dimsize>1</Dimsize><String><Name>String</Name><Val>M2L:3:9:1</Val></String></Array></Cluster><Cluster><Name>Alias</Name><NumElts>2</NumElts><String><Name>Name</Name><Val>dis_valve2</Val></String><Array><Name>Route</Name><Dimsize>1</Dimsize><String><Name>String</Name><Val>M2L:3:9:0</Val></String></Array></Cluster><Cluster><Name>Alias</Name><NumElts>2</NumElts><String><Name>Name</Name><Val>con_valve3</Val></String><Array><Name>Route</Name><Dimsize>1</Dimsize><String><Name>String</Name><Val>M2H:3:10:1</Val></String></Array></Cluster><Cluster><Name>Alias</Name><NumElts>2</NumElts><String><Name>Name</Name><Val>dis_valve3</Val></String><Array><Name>Route</Name><Dimsize>1</Dimsize><String><Name>String</Name><Val>M2H:3:10:0</Val></String></Array></Cluster><Cluster><Name>Alias</Name><NumElts>2</NumElts><String><Name>Name</Name><Val>con_valve4</Val></String><Array><Name>Route</Name><Dimsize>1</Dimsize><String><Name>String</Name><Val>M2L:3:10:1</Val></String></Array></Cluster><Cluster><Name>Alias</Name><NumElts>2</NumElts><String><Name>Name</Name><Val>dis_valve4</Val></String><Array><Name>Route</Name><Dimsize>1</Dimsize><String><Name>String</Name><Val>M2L:3:10:0</Val></String></Array></Cluster><Cluster><Name>Alias</Name><NumElts>2</NumElts><String><Name>Name</Name><Val>con_valve5</Val></String><Array><Name>Route</Name><Dimsize>1</Dimsize><String><Name>String</Name><Val>M2H:3:11:1</Val></String></Array></Cluster><Cluster><Name>Alias</Name><NumElts>2</NumElts><String><Name>Name</Name><Val>dis_valve5</Val></String><Array><Name>Route</Name><Dimsize>1</Dimsize><String><Name>String</Name><Val>M2H:3:11:0</Val></String></Array></Cluster><Cluster><Name>Alias</Name><NumElts>2</NumElts><String><Name>Name</Name><Val>con_valve6</Val></String><Array><Name>Route</Name><Dimsize>1</Dimsize><String><Name>String</Name><Val>M2L:3:11:1</Val></String></Array></Cluster><Cluster><Name>Alias</Name><NumElts>2</NumElts><String><Name>Name</Name><Val>dis_valve6</Val></String><Array><Name>Route</Name><Dimsize>1</Dimsize><String><Name>String</Name><Val>M2L:3:11:0</Val></String></Array></Cluster><Cluster><Name>Alias</Name><NumElts>2</NumElts><String><Name>Name</Name><Val>con_valve7</Val></String><Array><Name>Route</Name><Dimsize>1</Dimsize><String><Name>String</Name><Val>M2H:3:12:1</Val></String></Array></Cluster><Cluster><Name>Alias</Name><NumElts>2</NumElts><String><Name>Name</Name><Val>dis_valve7</Val></String><Array><Name>Route</Name><Dimsize>1</Dimsize><String><Name>String</Name><Val>M2H:3:12:0</Val></String></Array></Cluster><Cluster><Name>Alias</Name><NumElts>2</NumElts><String><Name>Name</Name><Val>con_valve8</Val></String><Array><Name>Route</Name><Dimsize>1</Dimsize><String><Name>String</Name><Val>M2L:3:12:1</Val></String></Array></Cluster><Cluster><Name>Alias</Name><NumElts>2</NumElts><String><Name>Name</Name><Val>dis_valve8</Val></String><Array><Name>Route</Name><Dimsize>1</Dimsize><String><Name>String</Name><Val>M2L:3:12:0</Val></String></Array></Cluster><Cluster><Name>Alias</Name><NumElts>2</NumElts><String><Name>Name</Name><Val>con_vdrain</Val></String><Array><Name>Route</Name><Dimsize>1</Dimsize><String><Name>String</Name><Val>M2H:3:13:1</Val></String></Array></Cluster><Cluster><Name>Alias</Name><NumElts>2</NumElts><String><Name>Name</Name><Val>dis_vdrain</Val></String><Array><Name>Route</Name><Dimsize>1</Dimsize><String><Name>String</Name><Val>M2H:3:13:0</Val></String></Array></Cluster><Cluster><Name>Alias</Name><NumElts>2</NumElts><String><Name>Name</Name><Val>con_vtemp</Val></String><Array><Name>Route</Name><Dimsize>1</Dimsize><String><Name>String</Name><Val>M2L:3:13:1</Val></String></Array></Cluster><Cluster><Name>Alias</Name><NumElts>2</NumElts><String><Name>Name</Name><Val>dis_vtemp</Val></String><Array><Name>Route</Name><Dimsize>1</Dimsize><String><Name>String</Name><Val>M2L:3:13:0</Val></String></Array></Cluster><Cluster><Name>Alias</Name><NumElts>2</NumElts><String><Name>Name</Name><Val>con_vpump</Val></String><Array><Name>Route</Name><Dimsize>1</Dimsize><String><Name>String</Name><Val>M2H:3:14:1</Val></String></Array></Cluster><Cluster><Name>Alias</Name><NumElts>2</NumElts><String><Name>Name</Name><Val>dis_vpump</Val></String><Array><Name>Route</Name><Dimsize>1</Dimsize><String><Name>String</Name><Val>M2H:3:14:0</Val></String></Array></Cluster><Cluster><Name>Alias</Name><NumElts>2</NumElts><String><Name>Name</Name><Val>con_vlarge</Val></String><Array><Name>Route</Name><Dimsize>1</Dimsize><String><Name>String</Name><Val>M2L:3:14:1</Val></String></Array></Cluster><Cluster><Name>Alias</Name><NumElts>2</NumElts><String><Name>Name</Name><Val>dis_vlarge</Val></String><Array><Name>Route</Name><Dimsize>1</Dimsize><String><Name>String</Name><Val>M2L:3:14:0</Val></String></Array></Cluster><Cluster><Name>Alias</Name><NumElts>2</NumElts><String><Name>Name</Name><Val>con_vsmall</Val></String><Array><Name>Route</Name><Dimsize>1</Dimsize><String><Name>String</Name><Val>M2H:3:15:1</Val></String></Array></Cluster><Cluster><Name>Alias</Name><NumElts>2</NumElts><String><Name>Name</Name><Val>dis_vsmall</Val></String><Array><Name>Route</Name><Dimsize>1</Dimsize><String><Name>String</Name><Val>M2H:3:15:0</Val></String></Array></Cluster><Cluster><Name>Alias</Name><NumElts>2</NumElts><String><Name>Name</Name><Val>con_pv1</Val></String><Array><Name>Route</Name><Dimsize>1</Dimsize><String><Name>String</Name><Val>M2L:3:15:1</Val></String></Array></Cluster><Cluster><Name>Alias</Name><NumElts>2</NumElts><String><Name>Name</Name><Val>dis_pv1</Val></String><Array><Name>Route</Name><Dimsize>1</Dimsize><String><Name>String</Name><Val>M2L:3:15:0</Val></String></Array></Cluster><Cluster><Name>Alias</Name><NumElts>2</NumElts><String><Name>Name</Name><Val>con_pv2</Val></String><Array><Name>Route</Name><Dimsize>1</Dimsize><String><Name>String</Name><Val>M2H:3:16:1</Val></String></Array></Cluster><Cluster><Name>Alias</Name><NumElts>2</NumElts><String><Name>Name</Name><Val>dis_pv2</Val></String><Array><Name>Route</Name><Dimsize>1</Dimsize><String><Name>String</Name><Val>M2H:3:16:0</Val></String></Array></Cluster><Cluster><Name>Alias</Name><NumElts>2</NumElts><String><Name>Name</Name><Val>con_fan</Val></String><Array><Name>Route</Name><Dimsize>1</Dimsize><String><Name>String</Name><Val>M2L:3:16:1</Val></String></Array></Cluster><Cluster><Name>Alias</Name><NumElts>2</NumElts><String><Name>Name</Name><Val>dis_fan</Val></String><Array><Name>Route</Name><Dimsize>1</Dimsize><String><Name>String</Name><Val>M2L:3:16:0</Val></String></Array></Cluster><Cluster><Name>Alias</Name><NumElts>2</NumElts><String><Name>Name</Name><Val>con_lcd_vcc</Val></String><Array><Name>Route</Name><Dimsize>1</Dimsize><String><Name>String</Name><Val>M2L:1:18:1</Val></String></Array></Cluster><Cluster><Name>Alias</Name><NumElts>2</NumElts><String><Name>Name</Name><Val>dis_lcd_vcc</Val></String><Array><Name>Route</Name><Dimsize>1</Dimsize><String><Name>String</Name><Val>M2L:1:18:0</Val></String></Array></Cluster><Cluster><Name>Alias</Name><NumElts>2</NumElts><String><Name>Name</Name><Val>con_adcin</Val></String><Array><Name>Route</Name><Dimsize>1</Dimsize><String><Name>String</Name><Val>M2H:1:19:1</Val></String></Array></Cluster><Cluster><Name>Alias</Name><NumElts>2</NumElts><String><Name>Name</Name><Val>dis_adcin</Val></String><Array><Name>Route</Name><Dimsize>1</Dimsize><String><Name>String</Name><Val>M2H:1:19:0</Val></String></Array></Cluster><Cluster><Name>Alias</Name><NumElts>2</NumElts><String><Name>Name</Name><Val>con_tp119</Val></String><Array><Name>Route</Name><Dimsize>1</Dimsize><String><Name>String</Name><Val>M2H:1:4:1</Val></String></Array></Cluster><Cluster><Name>Alias</Name><NumElts>2</NumElts><String><Name>Name</Name><Val>dis_tp119</Val></String><Array><Name>Route</Name><Dimsize>1</Dimsize><String><Name>String</Name><Val>M2H:1:4:0</Val></String></Array></Cluster><Cluster><Name>Alias</Name><NumElts>2</NumElts><String><Name>Name</Name><Val>con_button_led1</Val></String><Array><Name>Route</Name><Dimsize>1</Dimsize><String><Name>String</Name><Val>M2H:3:17:1</Val></String></Array></Cluster><Cluster><Name>Alias</Name><NumElts>2</NumElts><String><Name>Name</Name><Val>dis_button_led1</Val></String><Array><Name>Route</Name><Dimsize>1</Dimsize><String><Name>String</Name><Val>M2H:3:17:0</Val></String></Array></Cluster><Cluster><Name>Alias</Name><NumElts>2</NumElts><String><Name>Name</Name><Val>con_button_led2</Val></String><Array><Name>Route</Name><Dimsize>1</Dimsize><String><Name>String</Name><Val>M2L:3:17:1</Val></String></Array></Cluster><Cluster><Name>Alias</Name><NumElts>2</NumElts><String><Name>Name</Name><Val>dis_button_led2</Val></String><Array><Name>Route</Name><Dimsize>1</Dimsize><String><Name>String</Name><Val>M2L:3:17:0</Val></String></Array></Cluster><Cluster><Name>Alias</Name><NumElts>2</NumElts><String><Name>Name</Name><Val>con_button_led3</Val></String><Array><Name>Route</Name><Dimsize>1</Dimsize><String><Name>String</Name><Val>M2H:3:18:1</Val></String></Array></Cluster><Cluster><Name>Alias</Name><NumElts>2</NumElts><String><Name>Name</Name><Val>dis_button_led3</Val></String><Array><Name>Route</Name><Dimsize>1</Dimsize><String><Name>String</Name><Val>M2H:3:18:0</Val></String></Array></Cluster></Array></Config>"
  out "Config":T2
  # "Row:Column: State ie R10:C2:1"
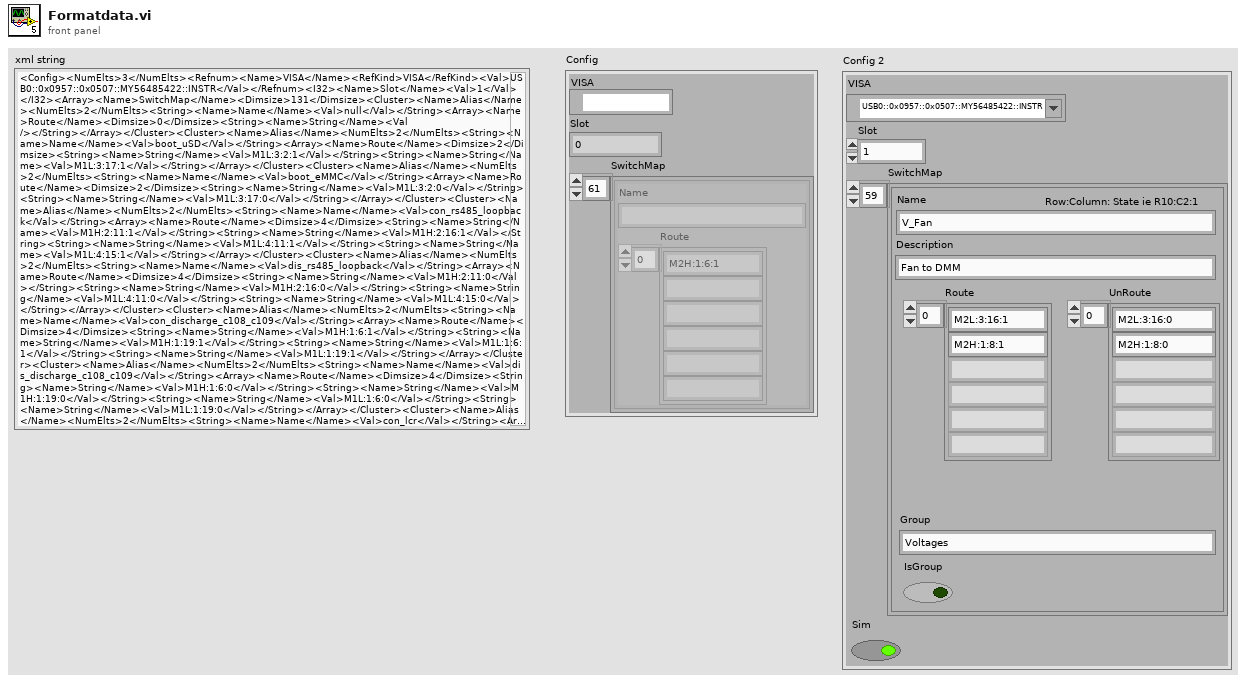
[diagram p1: front panel]
types:
  T1 = cluster{"VISA":refnum<visa-resource-name>, "Slot":i32, "SwitchMap":cluster{"Name":string, "Route":string[], "UnRoute":string[], "Description":string, "Group":string, "IsGroup":bool}[], "Sim":bool}
  T2 = cluster{"VISA":refnum<visa-resource-name>, "Slot":i32, "SwitchMap":cluster{"Name":string, "Route":string[]}[]}
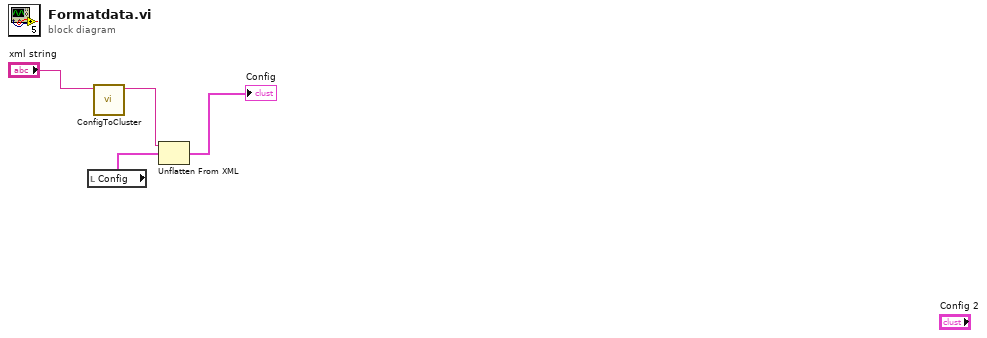
[diagram p0: block diagram]
diagram:
  n1 = local read "Config"() -> (w4:T2)
  n2 = call "ConfigToCluster.vi"("Config XML"="xml string") -> ("Cluster XML"=w1:string)  [unwired: 10 in]
  n3 = Unflatten From XML(xml string=w1, type=w4) -> (value=→"Config":T2)  [unwired: 1 in, 1 out]
